vi "Msg.vi"(7 "Actor in":refnum<class "Actor.lvclass">, 11 "Panel Create Msg in":refnum<class "Panel Create Msg.lvclass">) -> (5 "Actor out":refnum<class "Actor.lvclass">)   [LabVIEW 2021, in "Panel Create.lvlib" / "Panel Create Msg.lvclass"]
uses:
  Panel Create Msg.lvclass
  <vilib>/jettl/jettl/Actor/Actor/Actor.lvclass
  Panel Create/Panel Create.lvclass
  ddbfa231-e8ee-4a3e-88a9-b02c1223271b.vi
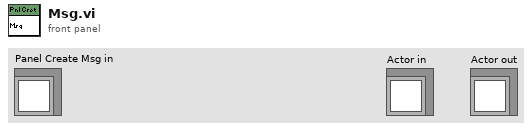
[diagram p1: front panel]
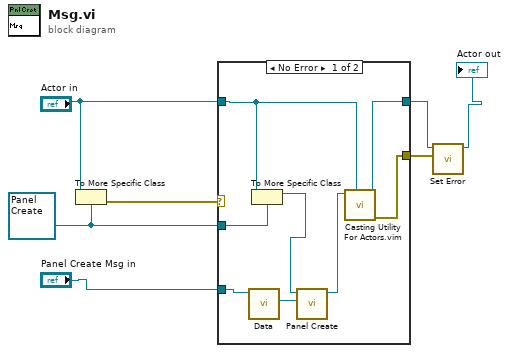
[diagram p0: block diagram]
diagram:
  w4 = refnum<class "Panel Create.lvclass"> refnum ("Panel Create.lvlib:Panel Create.lvclass")
  n1 = To More Specific Class(target class=w4, reference="Actor in") -> (error out=w7:errorcluster)  [unwired: 1 in, 1 out]
  n2 = case shown="No Error" w7 {
    selector: w7 -> [_ w16]
    tunnel: [w14 w17] -> w6
    tunnel: "Actor in" -> [w13 w17]
    tunnel: w4 -> [w15 _]
    tunnel: "Panel Create Msg in" -> [w11 _]
    tunnel: [w12 w16] -> w5
    frame No Error {
      n3 = call "Data.vi"("Panel Create Msg in"=w11) -> ("Panel"=w9:refnum<class "Panel.lvclass">)  [unwired: 10 in]
      n4 = To More Specific Class(target class=w15, reference=w13) -> (specific class reference=w10:refnum<class "Panel Create.lvclass">)  [unwired: 1 in, 1 out]
      n5 = call-dynamic "Panel Create.vi"("Panel"=w9, "Panel Create in"=w10) -> ("Panel Create out"=w8:refnum<class "Panel Create.lvclass">)  [unwired: 9 in]
      n6 = call "Casting Utility For Actors.vim"("type"=w13, "Actor in"=w8) -> ("error out"=w12:errorcluster, "Actor out"=w14:refnum<class "Actor.lvclass">)  [unwired: 8 in]
    }
    frame Error {
    }
  }
  n7 = call-dynamic "Set Error.vi"("Error"=w5, "Set Error in"=w6) -> ("Set Error out"=→"Actor out":refnum<class "Actor.lvclass">)  [unwired: 9 in]
